vi "Main.vi"() -> ()   [LabVIEW 2023]
doc: "This template is for the Queued Message Handler design pattern.\n\nThe Event Handling Loop generates messages based on user interface actions.\n\nThe Message Handling Loop processes messages generated by the Event Handling Loop, or by other messages. The messages are string values, so new messages can be added easily to the Message Cases case structure in the Message Handling Loop. Each message cluster can also provide an optional value for Message Data, which is a variant that can be converted to whatever message-specific data is required."
uses:
  controls/UI Data.ctl
  support/Message Queue/Enqueue Message (Single).vi
  <vilib>/Utility/error.llb/Error Cluster From Error Code.vi
  <vilib>/ErrorRing/Error Ring.xnode
  support/Message Queue/Message Queue.lvlib
  support/User Event - Stop/User Event - Stop.lvlib
panel:
  out "Action":bool
  out "Display <Replace Me>":string
  in  "Do Something Else <Replace Me>":bool
  in  "Do Something <Replace Me>":bool
  in  "Exit":bool
  # "These controls have associated \"Value Changed\" events configured in the Event Structure on the diagram.\n\nReplace them (and reconfigure the Event Structure) with the controls you need for your application."
  # "This template is for the Queued Message Handler design pattern.\n\nSee the block diagram for more information on how to use this template."
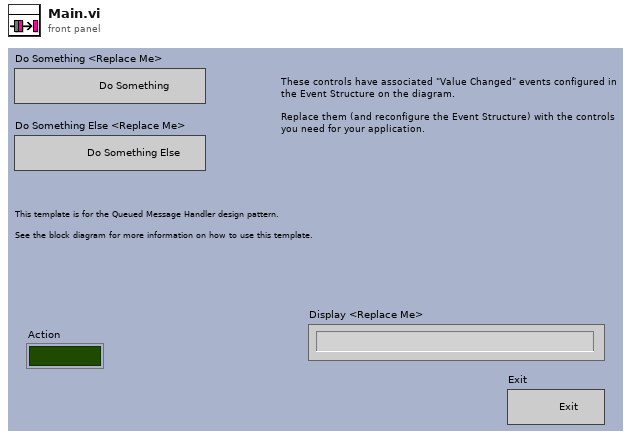
[diagram p1: front panel]
types:
  T1 = typedef "UI Data.ctl" = cluster{"Boolean <Replace Me>":bool, "String <Replace Me>":string, "Numeric <Replace Me>":dbl, "Do Something Ref":refnum<vi>, "Do Something Else Ref":refnum<vi>, "Data Display Ref":refnum<vi>, "Exit Button Ref":refnum<vi>}
  T2 = typedef "Message Queue.lvlib/All Message Queues.ctl" = cluster{"UI":refnum<queue>}
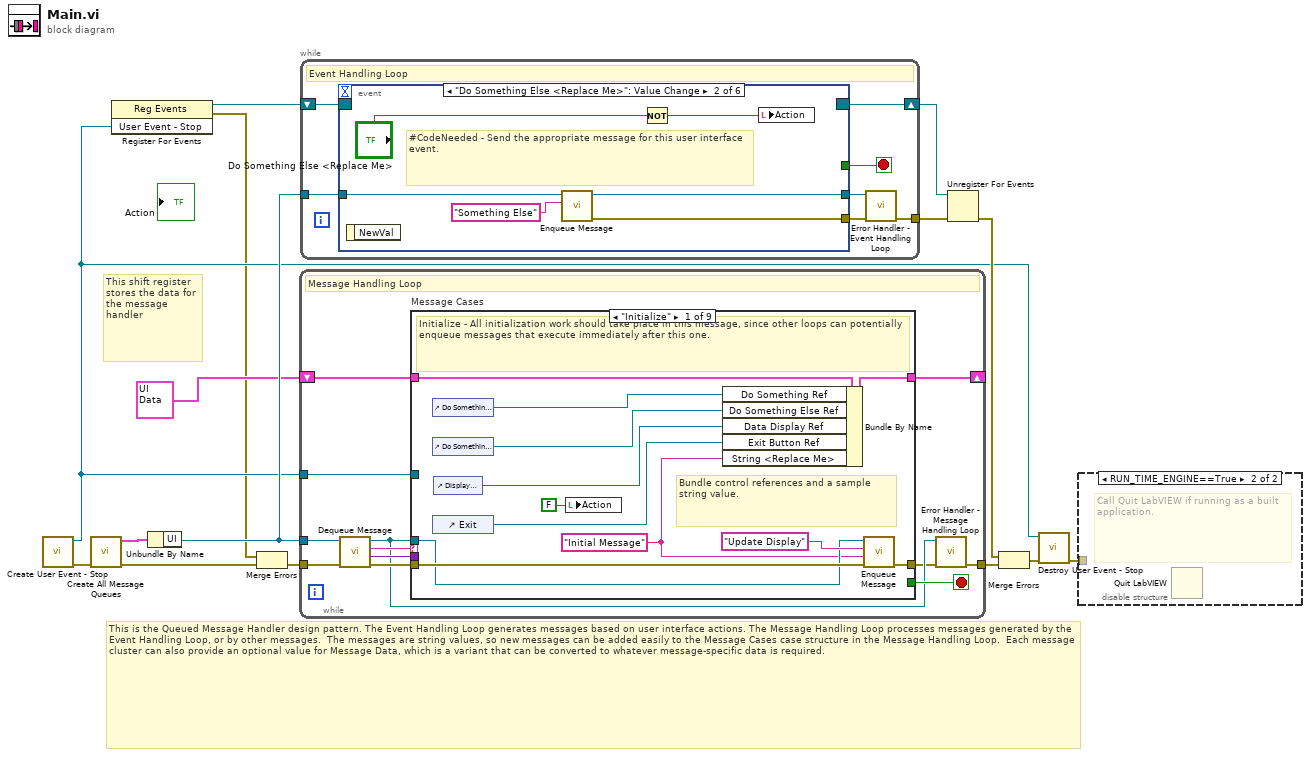
[diagram p0: block diagram]
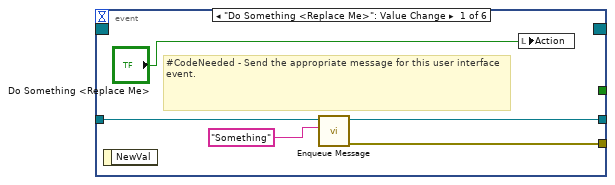
[diagram p3: hidden frame]
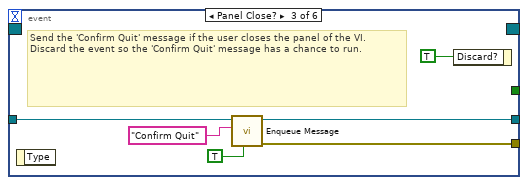
[diagram p4: hidden frame]
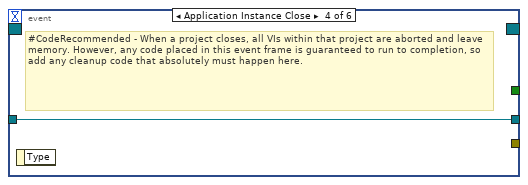
[diagram p5: hidden frame]
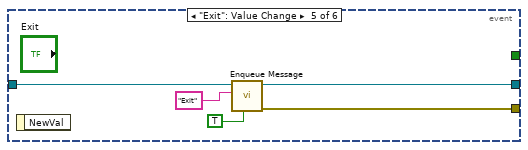
[diagram p6: hidden frame]
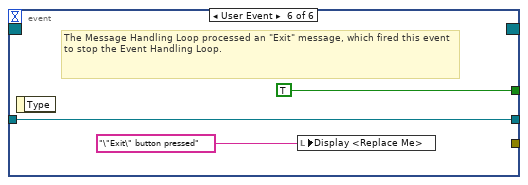
[diagram p7: hidden frame]
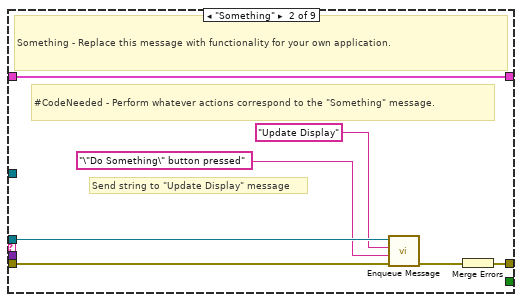
[diagram p8: hidden frame]
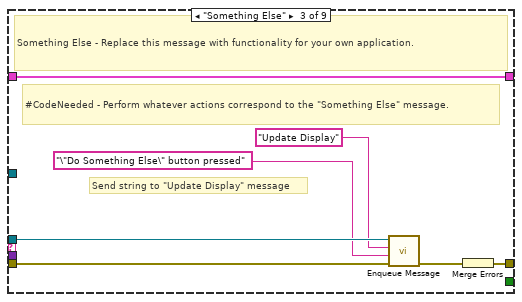
[diagram p9: hidden frame]
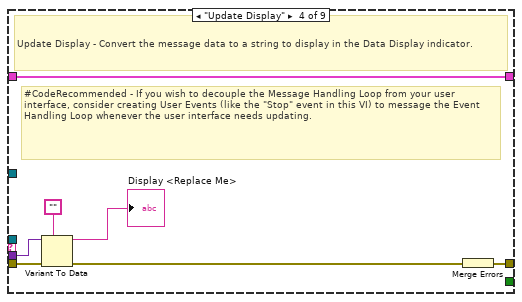
[diagram p10: hidden frame]
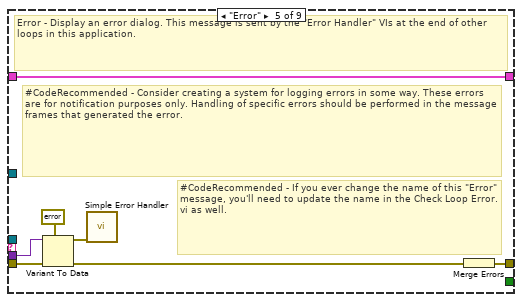
[diagram p11: hidden frame]
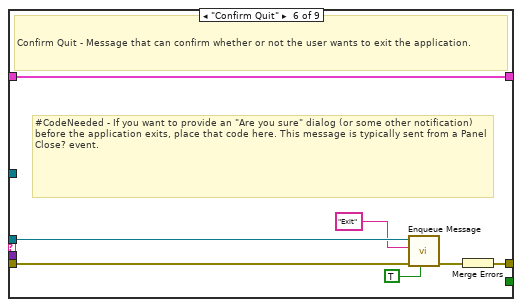
[diagram p12: hidden frame]
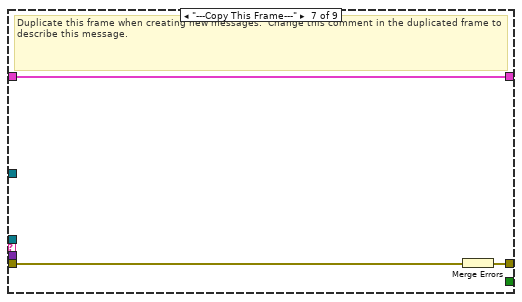
[diagram p13: hidden frame]
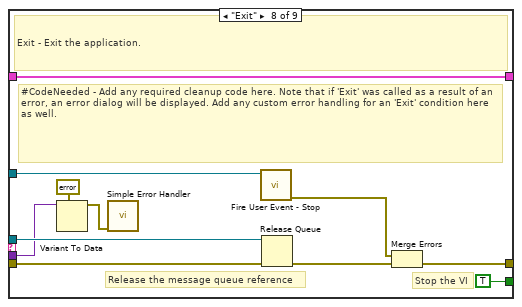
[diagram p14: hidden frame]
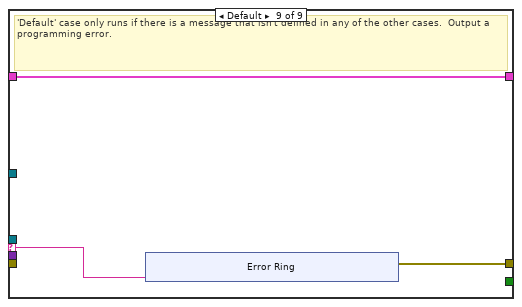
[diagram p15: hidden frame]
diagram:
  # "This is the Queued Message Handler design pattern. The Event Handling Loop generates messages based on user interface actions. The Message Handling Loop processes messages generated by the Event Handling Loop, or by other messages.  The messages are string values, so new messages can be added easily to the Message Cases case structure in the Message Handling Loop.  Each message cluster can also provide an optional value for Message Data, which is a variant that can be converted to whatever message-specific data is required."
  # "This shift register stores the data for the message handler"
  n1 = call "Create User Event - Stop.vi"() -> ("error out"=w11:errorcluster, "User Event - Stop"=w3:refnum<user-event>)  [unwired: 10 in]
  n2 = call "Create All Message Queues.vi"("error in (no error)"=w11) -> ("error out"=w15:errorcluster, "Message Queues out"=w14:T2)  [unwired: 9 in]
  n3 = register-events(w3) -> (reference out=w4:refnum<event-registration>, error out=w1:errorcluster)  [unwired: 2 in]
  n4 = Unbundle By Name(w14) -> ("UI"=w12:refnum<queue>)
  n5 = Merge Errors(w1, w15) -> (w2:errorcluster)
  n6 = while {
    tunnel: w12 -> [w19]
    shift-right: [w26] -> _
    shift-left: T1 {"Boolean <Replace Me>"=FALSE, "String <Replace Me>"="", "Numeric <Replace Me>"=0.0, "Do Something Ref"=refnum, "Do Something Else Ref"=refnum, "Data Display Ref"=refnum, "Exit Button Ref"=refnum} ("Data Cluster") -> [w27]
    tunnel: w3 -> [w24]
    tunnel: w2 -> [w23]
    tunnel: [w17] -> w13
    stop <- w25 stop-if-true
    # "Message Handling Loop"
    n7 = call "Dequeue Message.vi"("error in (no error)"=w23, "Message Queue"=w19) -> ("error out"=w22:errorcluster, "Message Data"=w20:variant, "Message"=w21:string, "dup Message Queue"=w18:refnum<queue>)  [unwired: 6 in]
    n8 = case "Message Cases" shown="\"Initialize\"" w21 {
      selector: w21 -> [_ _ _ _ _ _ _ _ w89]
      tunnel: w18 -> [w30 w42 w49 _ _ w70 _ w88 _]
      tunnel: w22 -> [w38 w44 w51 w58 w67 w74 w77 w81 _]
      tunnel: [w39 w45 w52 w59 w61 w72 w75 w84 w90] -> w16
      tunnel: w27 -> [w37 w46 w53 w60 w66 w73 w76 w87 w91]
      tunnel: [w36 w46 w53 w60 w66 w73 w76 w87 w91] -> w26
      tunnel: [_ _ _ _ _ _ _ TRUE _] -> w25
      tunnel: w20 -> [_ _ _ w57 w65 _ _ w78 _]
      tunnel: w24 -> [_ _ _ _ _ _ _ w83 _]
      frame "Initialize" {
        w29 = "Initial Message" ("Initial Message")
        # "Bundle control references and a sample string value."
        # "Initialize - All initialization work should take place in this message, since other loops can potentially enqueue messages that execute immediately after this one."
        n9 = control-ref of="Do Something <Replace Me>"() -> (w35:refnum<vi>)
        n10 = control-ref of="Do Something Else <Replace Me>"() -> (w34:refnum<vi>)
        n11 = control-ref of="Exit"() -> (w32:refnum<vi>)
        n12 = control-ref of="Display <Replace Me>"() -> (w33:refnum<vi>)
        n13 = local write "Action"(FALSE ("Action")) -> ()
        n14 = Bundle By Name(cluster=w37, "Do Something Ref"=w35, "Do Something Else Ref"=w34, "Data Display Ref"=w33, "Exit Button Ref"=w32, "String <Replace Me>"=w29) -> (w36:T1)
        n15 = call-poly "Enqueue Message.vi"("error in (no error)"=w38, "Message Data"=w29, "Message"="Update Display", "Message Queue"=w30) -> ("error out"=w39:errorcluster)  [unwired: 6 in, 1 out]
      }
      frame "Something" {
        # "Send string to \"Update Display\" message"
        # "#CodeNeeded - Perform whatever actions correspond to the \"Something\" message."
        # "Something - Replace this message with functionality for your own application."
        n16 = call-poly "Enqueue Message.vi"("error in (no error)"=w44, "Message Data"="\"Do Something\" button pressed" ("\"Do Something\" button pressed"), "Message"="Update Display", "Message Queue"=w42) -> ("error out"=w43:errorcluster)  [unwired: 6 in, 1 out]
        n17 = Merge Errors(w43) -> (w45:errorcluster)
      }
      frame "Something Else" {
        # "Send string to \"Update Display\" message"
        # "#CodeNeeded - Perform whatever actions correspond to the \"Something Else\" message."
        # "Something Else - Replace this message with functionality for your own application."
        n18 = call-poly "Enqueue Message.vi"("error in (no error)"=w51, "Message Data"="\"Do Something Else\" button pressed" ("\"Do Something Else\" button pressed"), "Message"="Update Display", "Message Queue"=w49) -> ("error out"=w50:errorcluster)  [unwired: 6 in, 1 out]
        n19 = Merge Errors(w50) -> (w52:errorcluster)
      }
      frame "Update Display" {
        # "#CodeRecommended - If you wish to decouple the Message Handling Loop from your user interface, consider creating User Events (like the \"Stop\" event in this VI) to message the Event Handling Loop whenever the user interface needs updating."
        # "Update Display - Convert the message data to a string to display in the Data Display indicator."
        n20 = Variant To Data(error in=w58, type="", Variant=w57) -> (data=→"Display <Replace Me>":string, error out=w55:errorcluster)
        n21 = Merge Errors(w55) -> (w59:errorcluster)
      }
      frame "Error" {
        # "#CodeRecommended - If you ever change the name of this \"Error\" message, you'll need to update the name in the Check Loop Error.vi as well."
        # "#CodeRecommended - Consider creating a system for logging errors in some way. These errors are for notification purposes only. Handling of specific errors should be performed in the message frames that generated the error."
        # "Error - Display an error dialog. This message is sent by the \"Error Handler\" VIs at the end of other loops in this application."
        n22 = Variant To Data(error in=w67, type=errorcluster {"status"=FALSE, "code"=0, "source"=""} ("error constant"), Variant=w65) -> (data=w63:errorcluster, error out=w62:errorcluster)
        n23 = call <vilib>:"Simple Error Handler.vi"("error in (no error)"=w63) -> ()  [unwired: 4 in, 5 out]
        n24 = Merge Errors(w62) -> (w61:errorcluster)
      }
      frame "Confirm Quit" {
        # "#CodeNeeded - If you want to provide an \"Are you sure\" dialog (or some other notification) before the application exits, place that code here. This message is typically sent from a Panel Close? event."
        # "Confirm Quit - Message that can confirm whether or not the user wants to exit the application."
        n25 = call-poly "Enqueue Message.vi"("Priority Message? (F)"=TRUE, "error in (no error)"=w74, "Message"="Exit", "Message Queue"=w70) -> ("error out"=w71:errorcluster)  [unwired: 6 in, 1 out]
        n26 = Merge Errors(w71) -> (w72:errorcluster)
      }
      frame "---Copy This Frame---" {
        # "Duplicate this frame when creating new messages.  Change this comment in the duplicated frame to describe this message."
        n27 = Merge Errors(w77) -> (w75:errorcluster)
      }
      frame "Exit" {
        # "Stop the VI"
        # "Release the message queue reference"
        # "#CodeNeeded - Add any required cleanup code here. Note that if 'Exit' was called as a result of an error, an error dialog will be displayed. Add any custom error handling for an 'Exit' condition here as well."
        # "Exit - Exit the application."
        n28 = Variant To Data(type=errorcluster {"status"=FALSE, "code"=0, "source"=""} ("error constant"), Variant=w78) -> (data=w79:errorcluster)  [unwired: 1 in, 1 out]
        n29 = call <vilib>:"Simple Error Handler.vi"("error in (no error)"=w79) -> ()  [unwired: 4 in, 5 out]
        n30 = call "Fire User Event - Stop.vi"("User Event - Stop"=w83) -> ("error out"=w82:errorcluster)  [unwired: 10 in]
        n31 = Release Queue(queue=w88, error in (no error)=w81) -> (error out=w85:errorcluster)  [unwired: 1 in, 2 out]
        n32 = Merge Errors(w82, w85) -> (w84:errorcluster)
      }
      frame Default {
        # "'Default' case only runs if there is a message that isn't defined in any of the other cases.  Output a programming error."
        n33 = xnode "Error Ring"("parameter 0"=w89) -> ("error out"=w90:errorcluster)
      }
    }
    n34 = call "Error Handler - Message Handling Loop.vi"("error in (no error)"=w16, "Message Queue"=w18) -> ("dup error in"=w17:errorcluster)  [unwired: 8 in, 1 out]
  }
  n35 = while {
    tunnel: w12 -> [w105]
    shift-right: [w103] -> w8
    shift-left: w4 -> [w104]
    tunnel: [w99] -> w5
    stop <- w101 stop-if-true
    # "Event Handling Loop"
    n36 = event shown="[1] \"Do Something Else <Replace Me>\": Value Change" {
      selector: w104 -> [_ _ _ _ _ _]
      dyn-events: [_ _ _ _ _ _] -> w103
      timeout: _ -> [_ _ _ _ _ _]
      tunnel: [_ _ _ _ _ TRUE ("Discard?")] -> w101
      tunnel: w105 -> [w110 w116 w121 w123 w128 w131]
      tunnel: [w107 w113 w120 _ w127 _] -> w102
      tunnel: [w109 w115 w119 w123 w126 w131] -> w100
      event "Do Something <Replace Me>": Value Change {
        # "#CodeNeeded - Send the appropriate message for this user interface event."
        n37 = event-data() -> ()  [unwired: 1 in, 1 out]
        n38 = call-poly "Enqueue Message.vi"("Message"="Something", "Message Queue"=w110) -> ("error out"=w107:errorcluster, "dup Message Queue"=w109:refnum<queue>)  [unwired: 8 in]
        n39 = local write "Action"("Do Something <Replace Me>") -> ()
      }
      event "Do Something Else <Replace Me>": Value Change {
        # "#CodeNeeded - Send the appropriate message for this user interface event."
        n40 = event-data() -> ()  [unwired: 1 in, 1 out]
        n41 = call-poly "Enqueue Message.vi"("Message"="Something Else", "Message Queue"=w116) -> ("error out"=w113:errorcluster, "dup Message Queue"=w115:refnum<queue>)  [unwired: 8 in]
        n42 = Not(x="Do Something Else <Replace Me>") -> (.not. x?=w111:bool)
        n43 = local write "Action"(w111) -> ()
      }
      event Panel Close? {
        # "Send the 'Confirm Quit' message if the user closes the panel of the VI. Discard the event so the 'Confirm Quit' message has a chance to run."
        n44 = event-data() -> ()  [unwired: 1 in, 1 out]
        n45 = call-poly "Enqueue Message.vi"("Priority Message? (F)"=TRUE, "Message"="Confirm Quit", "Message Queue"=w121) -> ("error out"=w120:errorcluster, "dup Message Queue"=w119:refnum<queue>)  [unwired: 7 in]
        n46 = event-data("Discard?"=TRUE) -> ()  [unwired: 1 in, 1 out]
      }
      event Application Instance Close {
        # "#CodeRecommended - When a project closes, all VIs within that project are aborted and leave memory. However, any code placed in this event frame is guaranteed to run to completion, so add any cleanup code that absolutely must happen here."
        n47 = event-data() -> ()  [unwired: 1 in, 1 out]
      }
      event "Exit": Value Change {
        n48 = event-data() -> ()  [unwired: 1 in, 1 out]
        n49 = call-poly "Enqueue Message.vi"("Priority Message? (F)"=TRUE, "Message"="Exit", "Message Queue"=w128) -> ("error out"=w127:errorcluster, "dup Message Queue"=w126:refnum<queue>)  [unwired: 7 in]
      }
      event User Event {
        # "The Message Handling Loop processed an \"Exit\" message, which fired this event to stop the Event Handling Loop."
        n50 = event-data() -> ()  [unwired: 1 in, 1 out]
        n51 = local write "Display <Replace Me>"("\"Exit\" button pressed" ("VI Stopped")) -> ()
      }
    }
    n52 = call "Error Handler - Event Handling Loop.vi"("error in (no error)"=w102, "Message Queue"=w100) -> ("dup error in"=w99:errorcluster)  [unwired: 8 in, 1 out]
  }
  n53 = Unregister For Events(event registration refnum=w8, error in=w5) -> (error out=w9:errorcluster)
  n54 = Merge Errors(w9, w13) -> (w10:errorcluster)
  n55 = call "Destroy User Event - Stop.vi"("error in (no error)"=w10, "User Event - Stop"=w3) -> ("error out"=w6:errorcluster)  [unwired: 9 in]
  n56 = disable-structure shown="RUN_TIME_ENGINE==True" {
    disable-tunnel: w6 -> [_ _]
    frame condition #0 (active) {
    }
    frame condition #1 {
      # "Call Quit LabVIEW if running as a built application."
      n57 = Quit LabVIEW() -> ()  [unwired: 1 in]
    }
  }
